vi "verifyarrayCDB.vi"(2 "Array 2":cdb[](array[numeric]) format="%0.2f", 3 "Array 1":cdb[](array[numeric]) format="%0.2f", 4 "Master Array":cdb[](array[numeric]) format="%0.2f", 5 "Base":cdb format="%0.2f") -> (0 "Error Message":string, 1 "Success":bool=TRUE)   [LabVIEW 2012]
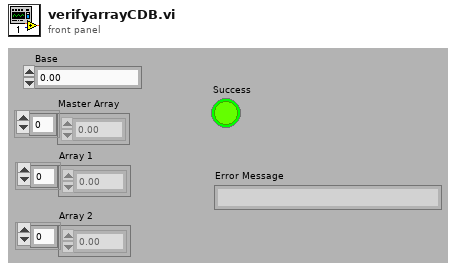
[diagram p1: front panel]
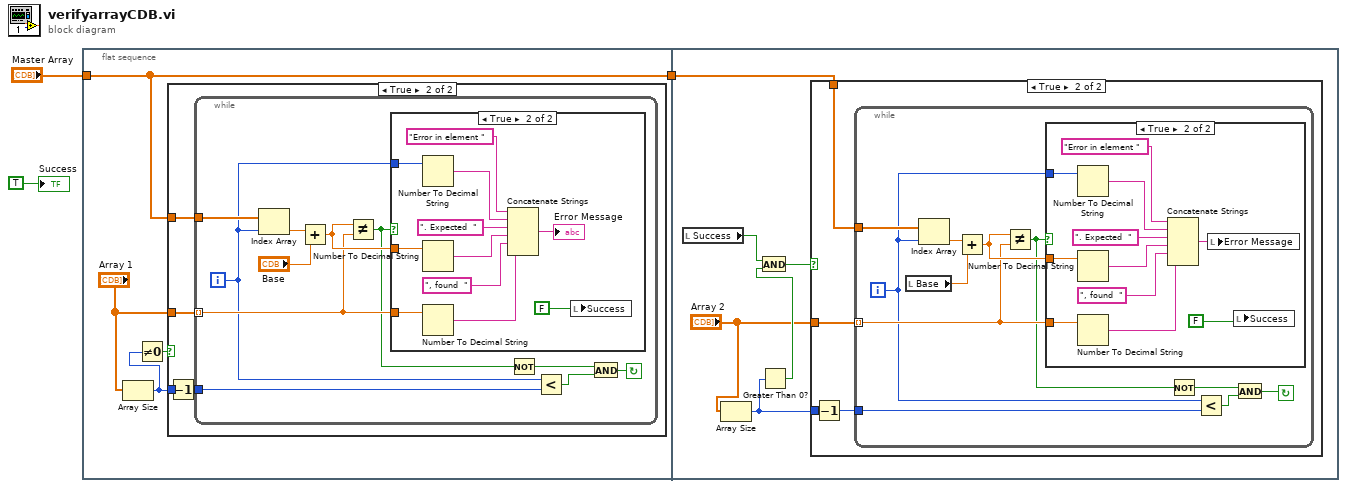
[diagram p0: block diagram]
diagram:
  n1 = flat-sequence {
    tunnel: "Master Array" -> [w6]
    tunnel: [w6] -> w2
    tunnel: w2 -> [w39]
    frame #0 {
      n2 = Array Size(array="Array 1") -> (size(s)=w4:i32)
      n3 = Not Equal To 0?(x=w4) -> (x != 0?=w5:bool)
      n4 = case shown="True" w5 {
        tunnel: "Array 1" -> [_ w11]
        tunnel: w4 -> [_ w10]
        tunnel: w6 -> [_ w9]
        frame False {
        }
        frame True {
          n5 = Decrement(x=w10) -> (x-1=w8:i32)
          n6 = while {
            tunnel: w11 -> [w18] mode=indexing
            tunnel: w9 -> [w22]
            tunnel: w8 -> [w16]
            i -> [w17]
            stop <- w12 continue-if-true
            n7 = Index Array(array=w22, index=w17) -> (element=w21:cdb)
            n8 = Add(x=w21, y="Base") -> (x+y=w19:cdb)
            n9 = Not Equal?(x=w19, y=w18) -> (x != y?=w14:bool)
            n10 = case shown="True" w14 {
              tunnel: w17 -> [_ w30]
              tunnel: w19 -> [_ w25]
              tunnel: w18 -> [_ w24]
              frame False {
              }
              frame True {
                n11 = Number To Decimal String(number=w30) -> (decimal integer string=w29:string)  [unwired: 1 out]
                n12 = Number To Decimal String(number=w25) -> (decimal integer string=w26:string)  [unwired: 1 out]
                n13 = Number To Decimal String(number=w24) -> (decimal integer string=w27:string)  [unwired: 1 out]
                n14 = Concatenate Strings("Error in element ", w29, ". Expected  ", w26, ", found  ", w27) -> (→"Error Message":string)
                n15 = local write "Success"(FALSE ("Success")) -> ()
              }
            }
            n16 = Not(x=w14) -> (.not. x?=w13:bool)
            n17 = Less?(x=w17, y=w16) -> (x < y?=w15:bool)
            n18 = And(x=w13, y=w15) -> (x .and. y?=w12:bool)
          }
        }
      }
    }
    frame #1 {
      n19 = local read "Success"() -> (w36:bool)
      n20 = Array Size(array="Array 2") -> (size(s)=w34:i32)
      n21 = Greater Than 0?(x=w34) -> (x > 0?=w37:bool)
      n22 = And(x=w36, y=w37) -> (x .and. y?=w38:bool)
      n23 = case shown="True" w38 {
        tunnel: w39 -> [_ w43]
        tunnel: w34 -> [_ w41]
        tunnel: "Array 2" -> [_ w40]
        frame False {
        }
        frame True {
          n24 = Decrement(x=w41) -> (x-1=w42:i32)
          n25 = while {
            tunnel: w40 -> [w51] mode=indexing
            tunnel: w43 -> [w54]
            tunnel: w42 -> [w49]
            i -> [w50]
            stop <- w45 continue-if-true
            n26 = local read "Base"() -> (w44:cdb)
            n27 = Index Array(array=w54, index=w50) -> (element=w53:cdb)
            n28 = Add(x=w53, y=w44) -> (x+y=w52:cdb)
            n29 = Not Equal?(x=w52, y=w51) -> (x != y?=w47:bool)
            n30 = case shown="True" w47 {
              tunnel: w50 -> [_ w62]
              tunnel: w52 -> [_ w58]
              tunnel: w51 -> [_ w57]
              frame False {
              }
              frame True {
                n31 = Number To Decimal String(number=w62) -> (decimal integer string=w61:string)  [unwired: 1 out]
                n32 = Number To Decimal String(number=w58) -> (decimal integer string=w59:string)  [unwired: 1 out]
                n33 = Number To Decimal String(number=w57) -> (decimal integer string=w60:string)  [unwired: 1 out]
                n34 = Concatenate Strings("Error in element ", w61, ". Expected  ", w59, ", found  ", w60) -> (w55:string)
                n35 = local write "Error Message"(w55) -> ()
                n36 = local write "Success"(FALSE ("Success")) -> ()
              }
            }
            n37 = Not(x=w47) -> (.not. x?=w46:bool)
            n38 = Less?(x=w50, y=w49) -> (x < y?=w48:bool)
            n39 = And(x=w46, y=w48) -> (x .and. y?=w45:bool)
          }
        }
      }
    }
  }
  "Success" <- TRUE ("Success")
